vi "Read With Abort.vi"(6 "abort":bool, 7 "timeout in ms (0)":i32, 10 "channel":T1) -> (2 "element":bool, 4 "aborted?":bool, 5 "missed":i32)   [LabVIEW 2020, in "Tag-bool.lvlib"]
doc: "Reads a value from a Tag channel or signals the channel to abort. This endpoint is the same as the Read endpoint except that it has an <B>abort</B> input and an <B>aborted?</B> output. You can use the abort capability of the Tag channel to close a channel abruptly, ignoring any data left in the channel buffer. You must use this endpoint together with the Write With Abort endpoint."
uses:
  <extravilib>/ChannelInstances/Tag-bool.lvlib
  <extravilib>/ChannelInstances/Tag-bool/))Channel.ctl
panel:
  # "number of values missed\n(-1 means element is stale or timed out)"
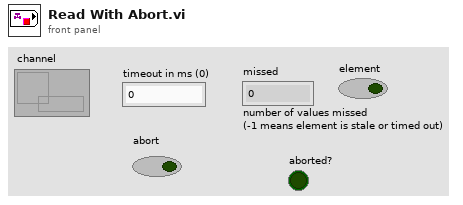
[diagram p1: front panel]
types:
  T1 = typedef "Tag-bool.lvlib/))Channel.ctl" = refnum<queue>
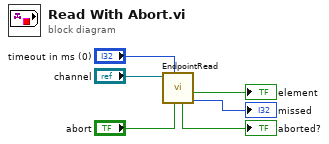
[diagram p0: block diagram]
diagram:
  n1 = call <extravilib>:"EndpointRead.vi"("abort (F)"="abort", "timeout in ms (-1)"="timeout in ms (0)", "channel in"="channel") -> ("missed"=→"missed":i32, "element out"=→"element":bool, "aborted?"=→"aborted?":bool)  [unwired: 5 in, 1 out]
